vi "Launch Nested Views.vi"(8 "error in (no error)":errorcluster, 9 "View Labels (optional)":string[](array[string]), 10 "Views":refnum<class "IViewable.lvclass">[](array[class]), 11 "IViewManager In":refnum<class "IViewManager.lvclass">) -> (0 "error out":errorcluster, 3 "IViewManager Out":refnum<class "IViewManager.lvclass">)   [LabVIEW 2015, in "IViewManager.lvlib" / "IViewManager.lvclass"]
doc: "<License>\nCopyright © 2017 Composed Systems, LLC | All rights reserved\nwww.composed.io\n\nAuthor: Ethan Stern <ethan.stern@composed.io>\n\nThis software is provided \"AS IS\" WITHOUT WARRANTIES, either express or implied, AND IS FOR EDUCATIONAL PURPOSES ONLY.\n</License>"
uses:
  IViewManager.lvclass
  IViewable/IViewable/IViewable.lvclass
  <vilib>/ActorFramework/Actor/Actor.lvclass/Actor.ctl
  <vilib>/ActorFramework/Message Enqueuer/Message Enqueuer.lvclass/Message Enqueuer.ctl
  IViewManager Messages/Populate Subpanels Msg/Populate Subpanels Msg.lvclass/Populate Subpanels Msg.ctl
  <vilib>/ActorFramework/Message Enqueuer/Init from Existing Queue.vi
  <vilib>/ActorFramework/Message Enqueuer/Enqueue.vi
  <vilib>/ActorFramework/Message Priority Queue/Priority Enqueue.vi
  <vilib>/ActorFramework/Message Enqueuer/Message Enqueuer.lvclass
  IViewManager Messages/Populate Subpanels Msg/Populate Subpanels Msg.lvclass
  <vilib>/ActorFramework/Actor/Actor.lvclass
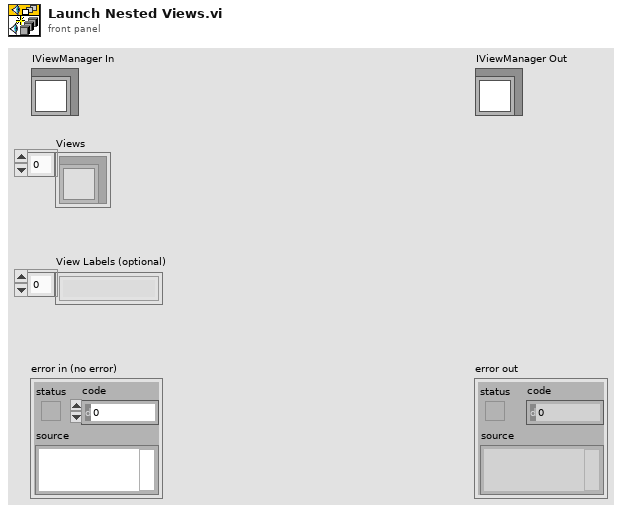
[diagram p1: front panel]
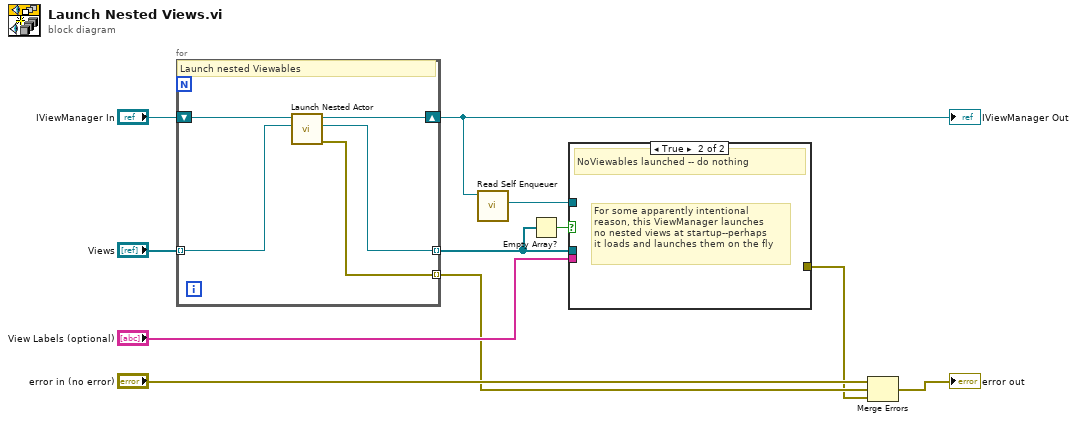
[diagram p0: block diagram]
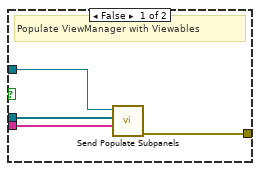
[diagram p2: hidden frame]
diagram:
  n1 = for {
    shift-right: [w15] -> w4
    shift-left: "IViewManager In" -> [w16]
    tunnel: "Views" -> [w14] mode=indexing
    tunnel: [w13] -> w2 mode=indexing
    tunnel: [w12] -> w6 mode=indexing
    # "Launch nested Viewables"
    n2 = call <vilib>:"Launch Nested Actor.vi"("Nested Actor"=w14, "Caller Actor in"=w16) -> ("error out"=w12:errorcluster, "Nested Actor's Enqueuer"=w13:refnum<class "Message Enqueuer.lvclass">, "Caller Actor out"=w15:refnum<class "IViewManager.lvclass">)  [unwired: 7 in]
  }
  "IViewManager Out" <- w4
  n3 = call <vilib>:"Read Self Enqueuer.vi"("Actor"=w4) -> ("Self Enqueuer"=w3:refnum<class "Message Enqueuer.lvclass">)  [unwired: 10 in]
  n4 = Empty Array?(array=w2) -> (empty?=w1:bool)
  n5 = case shown="True" w1 {
    tunnel: w2 -> [w20 _]
    tunnel: "View Labels (optional)" -> [w19 _]
    tunnel: [w18 _] -> w5
    tunnel: w3 -> [w17 _]
    frame False {
      # "Populate ViewManager with Viewables"
      n6 = call "Send Populate Subpanels.vi"("View Labels (optional)"=w19, "Views"=w20, "Message Enqueuer"=w17) -> ("error out"=w18:errorcluster)  [unwired: 7 in, 1 out]
    }
    frame True {
      # "For some apparently intentional\nreason, this ViewManager launches\nno nested views at startup--perhaps\nit loads and launches them on the fly"
      # "NoViewables launched -- do nothing"
    }
  }
  n7 = Merge Errors("error in (no error)", w6, w5) -> (→"error out":errorcluster)
